vi "Set Switch Heater.vi"(8 "error in (no error)":errorcluster, 10 "Switch Heater":T1, 11 "Instrument.1820 in":refnum<class "Instrument.OxfordVRM.lvclass">) -> (0 "error out":errorcluster, 2 "Response":string, 3 "Instrument.1820 in":refnum<class "Instrument.OxfordVRM.lvclass">)   [LabVIEW 2016, in "Instrument.OxfordVRM.lvclass"]
uses:
  Instrument.OxfordVRM.lvclass
  <instrlib>/Mercury iXX/Public/Libraries/Magnet/Controls/Switch Heater.ctl
  Typedefs/Instrument.Oxford1820.Commands-enum.ctl
  <instrlib>/Mercury iXX/Public/Libraries/Magnet.lvlib
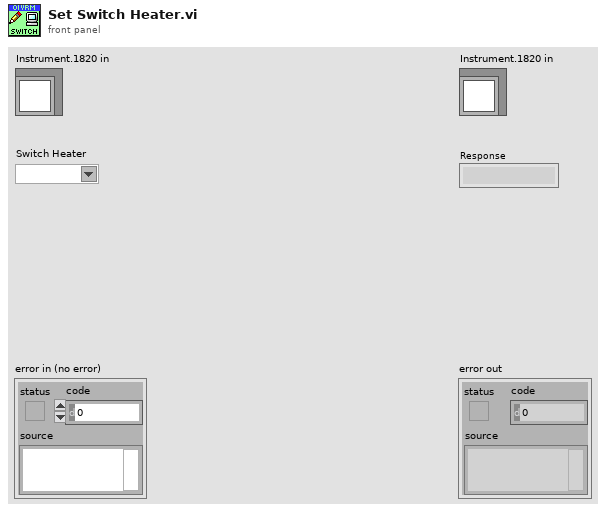
[diagram p1: front panel]
types:
  T1 = typedef "Mercury iXX.lvlib/Magnet.lvlib/Switch Heater.ctl" = string
  T2 = typedef "Instrument.OxfordVRM.lvclass/Instrument.Oxford1820.Commands-enum.ctl" = enum16{"setAction", "setTarget", "setSwitchHeat", "setLambda", "setFillMode", "setNeedleValve", "setMagnetField", "getStatus", "getTarget", "getSwitchHeat", "getPSUField", "newcommand", "getMagnetField"}
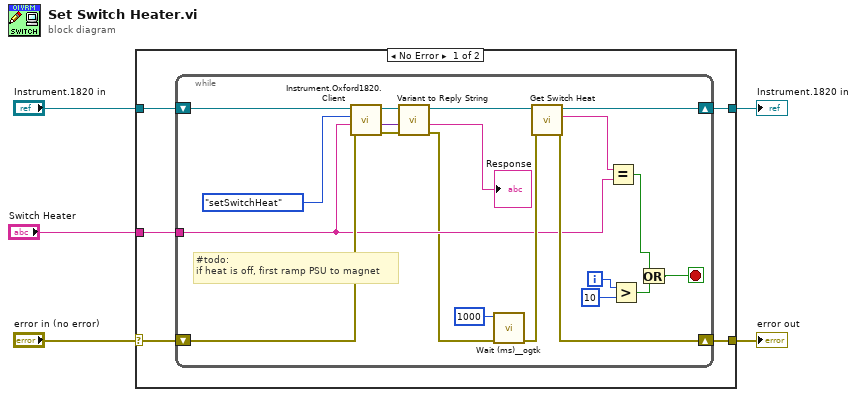
[diagram p0: block diagram]
diagram:
  n1 = case shown="No Error" "error in (no error)" {
    selector: "error in (no error)" -> [w9 w32]
    tunnel: [w8 w32] -> w4
    tunnel: [w7 w31] -> w2
    tunnel: "Instrument.1820 in" -> [w10 w31]
    tunnel: "Switch Heater" -> [w6 _]
    frame No Error {
      n2 = while {
        tunnel: w6 -> [w12]
        shift-right: [w28] -> w7
        shift-left: w10 -> [w23]
        shift-right: [w26] -> w8
        shift-left: w9 -> [w29]
        i -> [w18]
        stop <- w19 stop-if-true
        # "#todo:\nif heat is off, first ramp PSU to magnet"
        n3 = call "Instrument.Oxford1820.Client.vi"("error in (no error)"=w29, "Data"=w12, "Commands"=Instrument.Oxford1820.Commands-enum."setSwitchHeat", "Instrument.1820 in"=w23) -> ("error out"=w13:errorcluster, "Data out"=w14:variant, "Instrument.1820 out"=w16:refnum<class "Instrument.OxfordVRM.lvclass">)  [unwired: 5 in]
        n4 = call "Variant to Reply String.vi"("error in (no error)"=w13, "Data"=w14, "Instrument.1820 in"=w16) -> ("error out"=w11:errorcluster, "Reply"=→"Response":string, "Instrument.1820 out"=w15:refnum<class "Instrument.OxfordVRM.lvclass">)  [unwired: 6 in]
        n5 = call <userlib>:"Wait (ms)__ogtk.vi"("error in (no error)"=w11, "milliseconds to wait"=u32 1000) -> ("error out"=w25:errorcluster)  [unwired: 8 in, 1 out]
        n6 = call "Get Switch Heat.vi"("error in (no error)"=w25, "Instrument.1820 in"=w15) -> ("error out"=w26:errorcluster, "Switch Heater Status"=w27:string, "Instrument.1820 in"=w28:refnum<class "Instrument.OxfordVRM.lvclass">)  [unwired: 6 in, 1 out]
        n7 = Equal?(x=w27, y=w12) -> (x = y?=w20:bool)
        n8 = Greater?(x=w18, y=10) -> (0:w21:bool)
        n9 = Or(x=w20, y=w21) -> (x .or. y?=w19:bool)
      }
    }
    frame Error {
    }
  }
  "error out" <- w4
  "Instrument.1820 in" <- w2
